vi "Error Handler main loop.vi"(8 "error in (no error)":errorcluster, 10 "Exit?":bool, 11 "Queue in":refnum<queue>) -> (3 "Exit?":bool)   [LabVIEW 2015]
uses:
  TypeDefs/Queue Data.ctl
  App Data.vi
  App Strings.vi
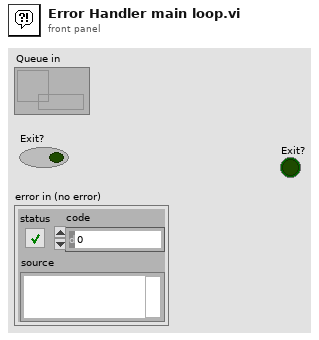
[diagram p1: front panel]
types:
  T1 = typedef "Queue Data.ctl" = cluster{"Action":string}
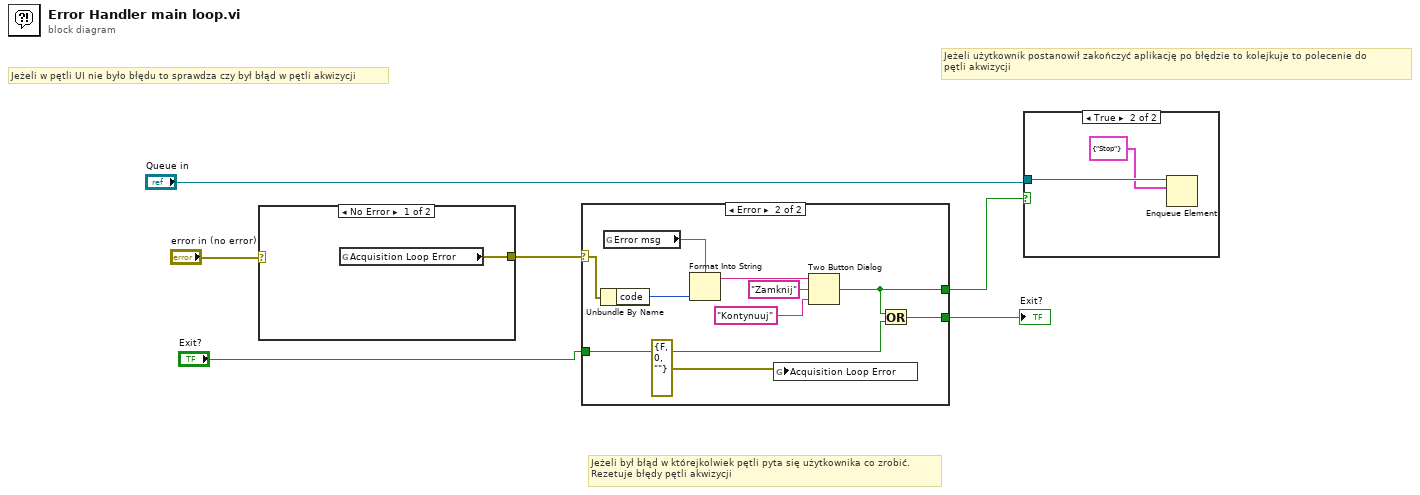
[diagram p0: block diagram]
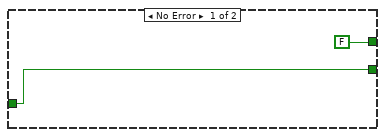
[diagram p3: hidden frame]
diagram:
  # "Jeżeli użytkownik postanowił zakończyć aplikację po błędzie to kolejkuje to polecenie do \npętli akwizycji"
  # "Jeżeli był błąd w którejkolwiek pętli pyta się użytkownika co zrobić.\nRezetuje błędy pętli akwizycji"
  # "Jeżeli w pętli UI nie było błędu to sprawdza czy był błąd w pętli akwizycji"
  n1 = case shown="No Error" "error in (no error)" {
    selector: "error in (no error)" -> [_ w8]
    tunnel: [w7 w8] -> w2
    frame No Error {
      n2 = global read "App Data.vi" "Acquisition Loop Error"() -> (w7:errorcluster)
    }
    frame Error {
    }
  }
  n3 = case shown="Error" w2 {
    selector: w2 -> [_ w19]
    tunnel: "Exit?" -> [w10 w14]
    tunnel: [w10 w13] -> w4
    tunnel: [FALSE w12] -> w6
    frame No Error {
    }
    frame Error {
      n4 = Unbundle By Name(w19) -> ("code"=w18:i32)
      n5 = global read "App Strings.vi" "Error msg"() -> (w20:string)
      n6 = Format Into String(format string=w20, w18) -> (resulting string=w17:string)  [unwired: 2 in, 1 out]
      n7 = global write "App Data.vi" "Acquisition Loop Error"(errorcluster {"status"=FALSE, "code"=0, "source"=""} ("Acquisition Loop Error")) -> ()
      n8 = Two Button Dialog(message=w17, 1:"Kontynuuj" ("T button name (\"OK\")"), 2:"Zamknij" ("T button name (\"OK\")")) -> (T button?=w12:bool)
      n9 = Or(x=w12, y=w14) -> (x .or. y?=w13:bool)
    }
  }
  "Exit?" <- w4
  n10 = case shown="True" w6 {
    tunnel: "Queue in" -> [_ w22]
    frame False {
    }
    frame True {
      n11 = Enqueue Element(queue=w22, element=T1 {"Action"="Stop"}) -> ()  [unwired: 2 in, 3 out]
    }
  }
